vi "timestamping.vi"() -> ()   [LabVIEW 2014]
panel:
  out "time stamp":timestamp
  in  "All Data":T1
  out "double precision float":dbl
  out "current time":timestamp
  in  "time format string (%c)":string
  out "date/time string":string
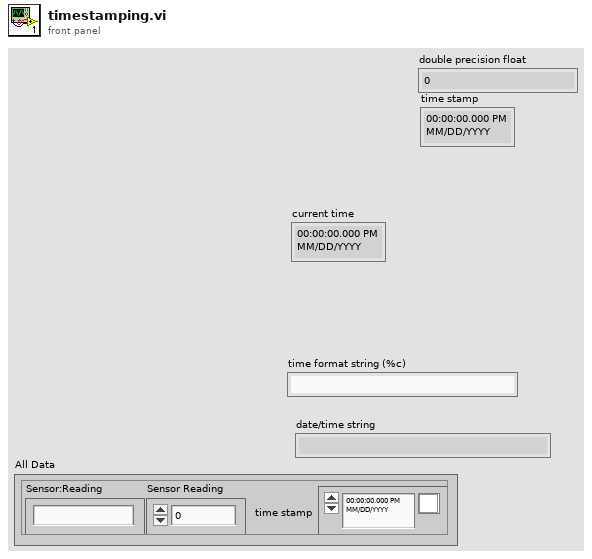
[diagram p1: front panel]
types:
  T1 = cluster{"Sensor:Reading":string, "Sensor Reading":dbl, "time stamp":timestamp}
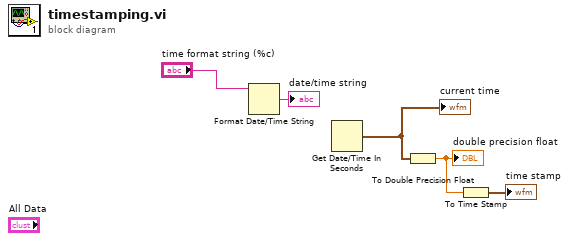
[diagram p0: block diagram]
diagram:
  n1 = Format Date/Time String(time format string (%c)="time format string (%c)") -> (date/time string=→"date/time string":string)  [unwired: 2 in]
  n2 = Get Date/Time In Seconds() -> (seconds since 1Jan1904=w3:timestamp)
  "current time" <- w3
  n3 = To Double Precision Float(number=w3) -> (double precision float=w2:dbl)
  "double precision float" <- w2
  n4 = To Time Stamp(1:w2) -> (0:→"time stamp":timestamp)
